vi "Main.vi"() -> ()   [LabVIEW 2023]
panel:
  in  "Sensor Type":string(combo)
  in  "AddSensor Button":bool
  in  "Sample time [s]":dbl=10.0
  in  "Exit":bool
  out "On/Off Light":bool
  in  "On/Off":bool
  out "Data Chart":dbl(graph)
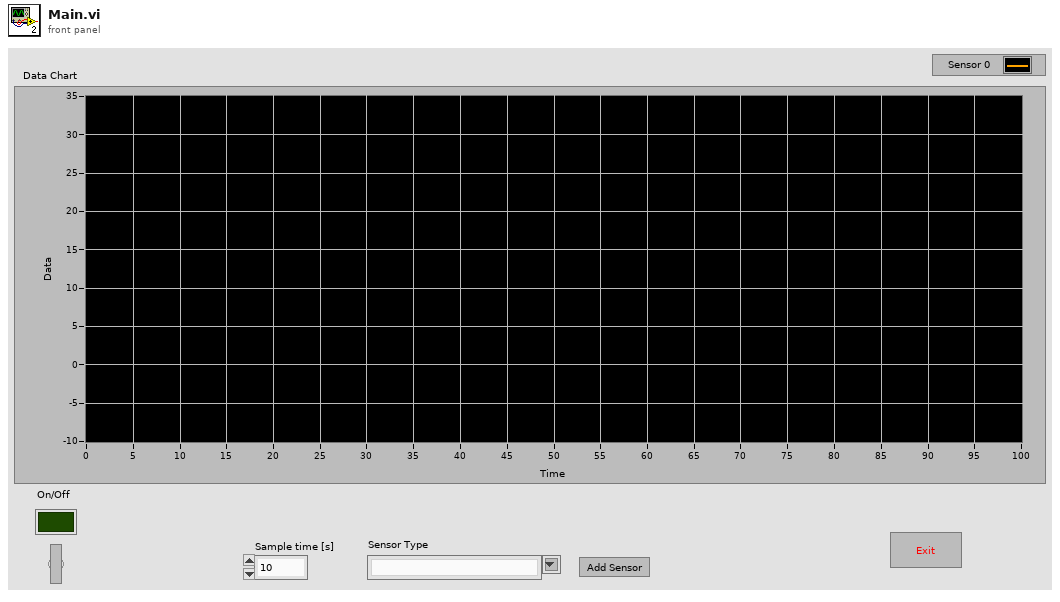
[diagram p1: front panel]
types:
  T1 = typedef "NI_Database_API.lvlib/Conn ObjectReference.ctl" = refnum<k1>
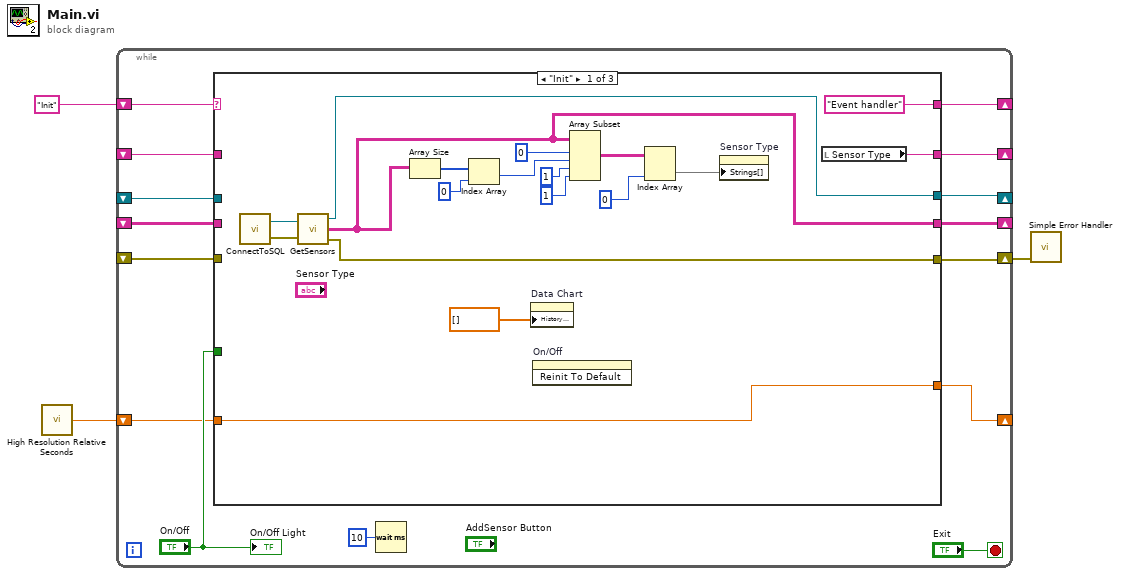
[diagram p0: block diagram]
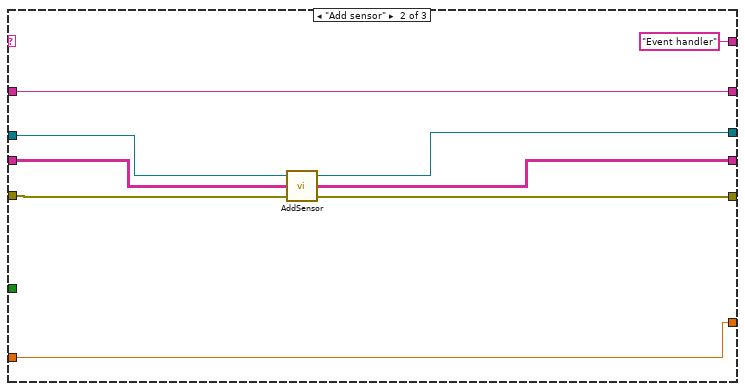
[diagram p2: hidden frame]
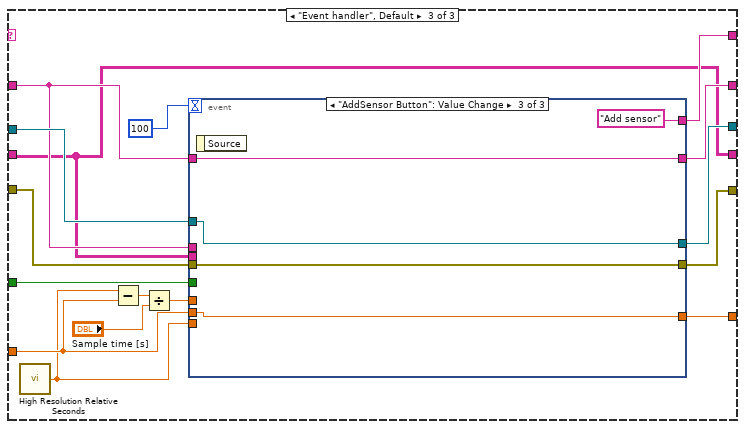
[diagram p3: hidden frame]
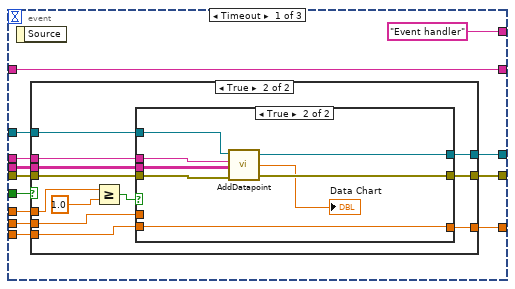
[diagram p4: hidden frame]
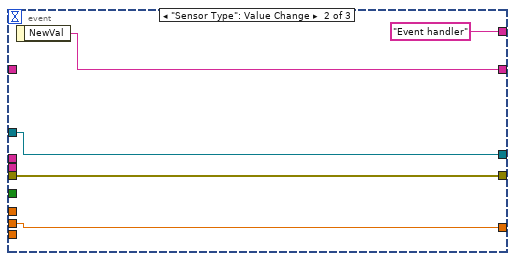
[diagram p7: hidden frame]
diagram:
  n1 = call <vilib>:"High Resolution Relative Seconds.vi"() -> ("relative seconds"=w1:dbl)
  n2 = while {
    shift-right: [w10] -> _
    shift-left: _ -> [w16]
    shift-right: [w15] -> _
    shift-left: "Init" -> [w17]
    shift-right: [w14] -> _
    shift-left: _ -> [w11]
    shift-right: [w13] -> w2
    shift-left: _ -> [w12]
    shift-right: [w7] -> _
    shift-left: w1 -> [w6]
    shift-right: [w5] -> _
    shift-left: _ -> [w4]
    stop <- "Exit" stop-if-true
    n3 = case shown="\"Init\"" w17 {
      tunnel: [w31 w41 w55] -> w13
      tunnel: w16 -> [_ w39 w48]
      tunnel: ["Event handler" "Event handler" w60] -> w15
      tunnel: [w29 w40 w56] -> w14
      tunnel: w12 -> [_ w43 w57]
      tunnel: w11 -> [_ w45 w58]
      tunnel: [w21 w39 w47] -> w10
      tunnel: "On/Off" -> [_ _ w59]
      tunnel: [w35 w42 w52] -> w7
      tunnel: w6 -> [w35 w42 w51]
      tunnel: [w20 w37 w46] -> w5
      tunnel: w4 -> [_ w38 w46]
      frame "Init" {
        n4 = call "ConnectToSQL.vi"() -> ("error out"=w32:errorcluster, "connection reference"=w33:T1)  [unwired: 2 in]
        n5 = call "GetSensors.vi"("connection reference"=w33, "error in (no error)"=w32) -> ("connection reference 2"=w29:T1, "data"=w20:string[][], "error out"=w31:errorcluster)
        n6 = Array Size(array=w20) -> (size(s)=w26:i32[])
        n7 = Index Array(array=w26, index=0) -> (element=w24:i32)
        n8 = property on="Data Chart" class="WFChart (strict)"("History Data"=dbl[] []) -> ()  [unwired: 2 in, 2 out]
        n9 = invoke on="On/Off" class="Bool (strict)" method="Reinit To Default"() -> ()  [unwired: 3 in, 3 out]
        n10 = Array Subset(array=w20, index (row)=0 ("index"), length (row)=w24, index (col)=1 ("index"), length (col)=1 ("length")) -> (w19:string[][])
        n11 = Index Array(array=w19, index (col)=0 ("dimension size")) -> (element=w22:string[])  [unwired: 1 in]
        n12 = property on="Sensor Type" class="CmbBox"("Strings[]"=w22) -> ()  [unwired: 2 in, 2 out]
        n13 = local read "Sensor Type"() -> (w21:string)
      }
      frame "Add sensor" {
        n14 = call "AddSensor.vi"("error in (no error)"=w43, "Sensors in"=w38, "connection reference in"=w45) -> ("error out"=w41:errorcluster, "Sensors out"=w37:string[][], "connection reference out"=w40:T1)
      }
      frame "Event handler", Default {
        n15 = call <vilib>:"High Resolution Relative Seconds.vi"() -> ("relative seconds"=w50:dbl)
        n16 = Subtract(x=w50, y=w51) -> (x-y=w54:dbl)
        n17 = Divide(x=w54, y="Sample time [s]") -> (x/y=w53:dbl)
        n18 = event shown="[2] \"AddSensor Button\": Value Change" {
          selector: _ -> [_ _ _]
          dyn-events: _ -> [_ _ _]
          timeout: 100 -> [_ _ _]
          tunnel: ["Event handler" "Event handler" "Add sensor"] -> w60
          tunnel: w59 -> [w73 _ _]
          tunnel: w58 -> [w72 w105 w108]
          tunnel: w57 -> [w71 w104 w109]
          tunnel: [w70 w105 w108] -> w56
          tunnel: [w69 w104 w109] -> w55
          tunnel: w48 -> [w68 _ _]
          tunnel: w53 -> [w67 _ _]
          tunnel: [w66 w102 w110] -> w52
          tunnel: w51 -> [w65 w102 w110]
          tunnel: w50 -> [w64 _ _]
          tunnel: [w63 w101 w106] -> w47
          tunnel: w48 -> [w63 _ w106]
          tunnel: w46 -> [w62 _ _]
          event Timeout {
            n19 = event-data() -> ()  [unwired: 1 in, 1 out]
            n20 = case shown="True" w73 {
              tunnel: w72 -> [w77 w89]
              tunnel: w71 -> [w76 w88]
              tunnel: [w77 w87] -> w70
              tunnel: [w76 w86] -> w69
              tunnel: w68 -> [_ w85]
              tunnel: w67 -> [_ w82]
              tunnel: [w75 w84] -> w66
              tunnel: w65 -> [w75 w83]
              tunnel: w64 -> [_ w79]
              tunnel: w62 -> [_ w78]
              frame False {
              }
              frame True {
                n21 = Greater Or Equal?(x=w82, y=1.0) -> (x >= y?=w81:bool)
                n22 = case shown="True" w81 {
                  tunnel: w89 -> [w91 w100]
                  tunnel: w88 -> [w90 w99]
                  tunnel: [w91 w98] -> w87
                  tunnel: [w90 w97] -> w86
                  tunnel: w85 -> [_ w94]
                  tunnel: [w92 w96] -> w84
                  tunnel: w83 -> [w92 _]
                  tunnel: w79 -> [_ w96]
                  tunnel: w78 -> [_ w93]
                  frame False {
                  }
                  frame True {
                    n23 = call "AddDatapoint.vi"("error in (no error)"=w99, "Sensor info"=w93, "Sensor Type"=w94, "connection reference in"=w100) -> ("error out"=w97:errorcluster, "Temperature"=→"Data Chart":dbl, "connection reference out"=w98:T1)
                  }
                }
              }
            }
          }
          event "Sensor Type": Value Change {
            n24 = event-data() -> ("NewVal"=w101:string)  [unwired: 1 in]
          }
          event "AddSensor Button": Value Change {
            n25 = event-data() -> ()  [unwired: 1 in, 1 out]
          }
        }
      }
    }
    n26 = Wait (ms)(milliseconds to wait=u32 10) -> ()  [unwired: 1 out]
    "On/Off Light" <- "On/Off"
  }
  n27 = call <vilib>:"Simple Error Handler.vi"("error in (no error)"=w2) -> ()  [unwired: 4 in, 5 out]
